vi "TDMS Reader.vi"() -> ()   [LabVIEW 2012]
panel:
  in  "数据集":u16(ring) items=["时间数据", "功率谱"]
  out "波形图":waveform(dbl)(graph)
  out "测试时间":timestamp=timestamp(-9593226000 s since 1904-01-01)
  out "测试操作员":string
  in  "序列号":string
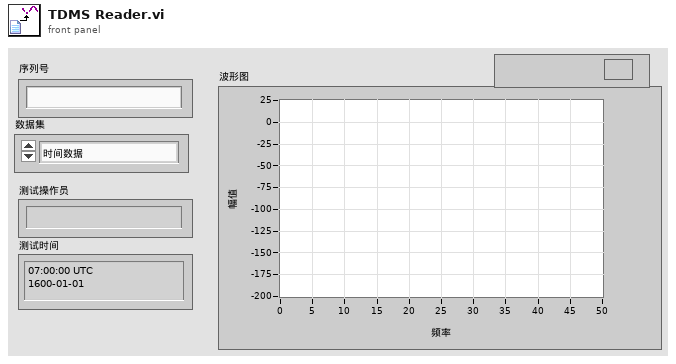
[diagram p1: front panel]
types:
  T1 = enum16{"open", "open or create", "create or replace", "create", "open (read-only)"}
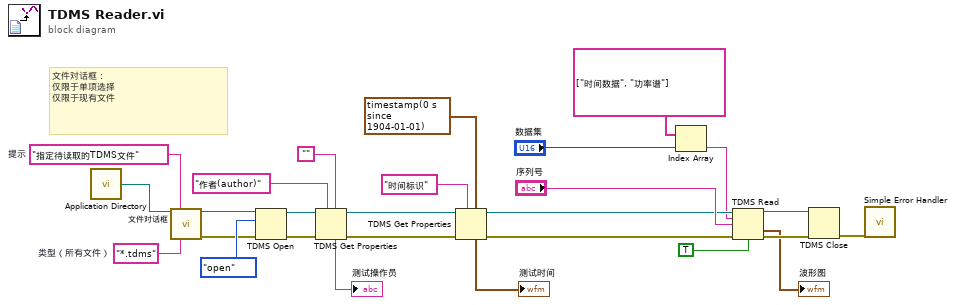
[diagram p0: block diagram]
diagram:
  w4 = "*.tdms"  # 类型（所有文件）
  w8 = "指定待读取的TDMS文件"  # 提示
  # "文件对话框：\n仅限于单项选择\n仅限于现有文件"
  n1 = call <vilib>:"Application Directory.vi"() -> ("Application Directory"=w7:path)
  n2 = call "文件对话框"("start path"=w7, "prompt"=w8, "pattern (all files)"=w4) -> ("selected path"=w5:path, "error out"=w6:errorcluster)  [unwired: 9 in, 2 out]
  n3 = TDMS Open ("TDMS打开")(8:w6, 10:T1."open" ("操作(0:open)"), 11:w5) -> (0:w22:errorcluster, 3:w23:refnum<k34>)  [unwired: 3 in]
  n4 = TDMS Get Properties ("TDMS获取属性")(5:"" ("空字符串常量"), 7:"作者(author)" ("属性名称"), 8:w22, 11:w23) -> (0:w19:errorcluster, 3:w21:refnum<k34>, 4:→"测试操作员":string)  [unwired: 5 out]
  n5 = TDMS Get Properties ("TDMS获取属性")(5:timestamp(0 s since 1904-01-01), 7:"时间标识" ("属性名称"), 8:w19, 11:w21) -> (0:w18:errorcluster, 3:w20:refnum<k34>, 4:→"测试时间":timestamp)  [unwired: 5 out]
  n6 = Index Array ("索引数组")(array=string[] ["时间数据", "功率谱"], index="数据集") -> (element=w1:string)
  n7 = TDMS Read ("TDMS读取")(0:w20, 5:w1, 7:"序列号", 11:w18, 13:TRUE ("按文件顺序返回通道？(F)")) -> (4:w25:refnum<k34>, 10:→"波形图":waveform(dbl), 15:w11:errorcluster)  [unwired: 3 in, 3 out]
  n8 = TDMS Close ("TDMS关闭")(8:w11, 11:w25) -> (0:w24:errorcluster)  [unwired: 1 out]
  n9 = call <vilib>:"Simple Error Handler.vi"("error in (no error)"=w24) -> ()  [unwired: 1 in, 8 out]
